vi "Untitled 1.vi"() -> ()   [LabVIEW 2013]
panel:
  in  "stop":bool
  out "theta":sgl(graph)
  in  "tsample":sgl
  in  "w":sgl
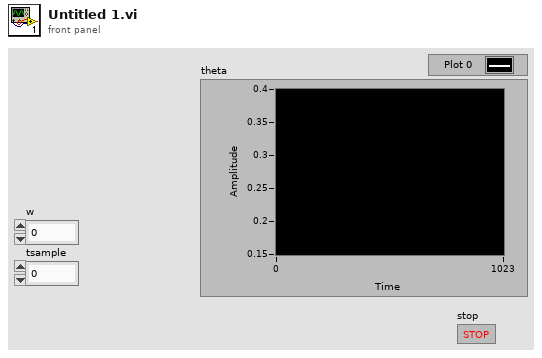
[diagram p1: front panel]
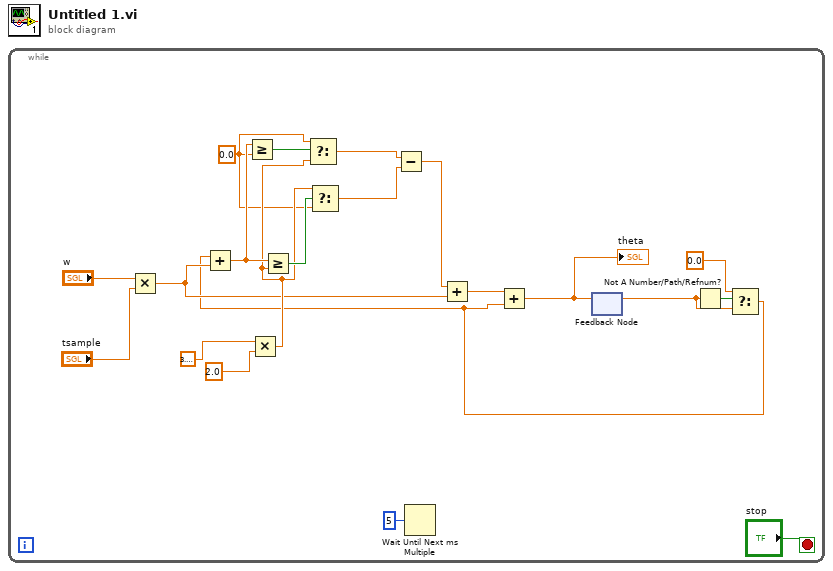
[diagram p0: block diagram]
diagram:
  n1 = while {
    stop <- "stop" stop-if-true
    w14 = sgl 0.0 ("y")
    n2 = Multiply(x="w", y="tsample") -> (x*y=w10:sgl)
    n3 = Multiply(x=sgl 3.1415927, y=sgl 2.0) -> (x*y=w15:sgl)
    n4 = Wait Until Next ms Multiple(millisecond multiple=u32 5) -> ()  [unwired: 1 out]
    n5 = feedback #1() -> (w4:sgl)  [unwired: 1 in]
    n6 = Not A Number/Path/Refnum?(number/path/refnum=w4) -> (NaN/Path/Refnum?=w7:bool)
    n7 = Select(t=sgl 0.0, s=w7, f=w4) -> (s? t:f=w3:sgl)
    n8 = Add(x=w3, y=w10) -> (x+y=w17:sgl)
    n9 = Greater Or Equal?(x=w17, y=w14) -> (x >= y?=w18:bool)
    n10 = Greater Or Equal?(x=w17, y=w15) -> (x >= y?=w19:bool)
    n11 = Select(t=w14, s=w18, f=w15) -> (s? t:f=w13:sgl)
    n12 = Select(t=w15, s=w19, f=w14) -> (s? t:f=w12:sgl)
    n13 = Subtract(x=w13, y=w12) -> (x-y=w11:sgl)
    n14 = Add(x=w11, y=w10) -> (x+y=w9:sgl)
    n15 = Add(x=w9, y=w3) -> (x+y=w5:sgl)
    "theta" <- w5
    n16 = feedback-in #1(w5) -> ()
  }
